vi "Find Var.vi"(8 "error in (no error)":errorcluster, 9 "Tag":string, 10 "Abs_Type Default":refnum<class "Abs_Type.lvclass">, 11 "Var Bus in":refnum<class "Var Bus.lvclass">) -> (0 "error out":errorcluster, 2 "Abs_Type Found":refnum<class "Abs_Type.lvclass">, 3 "Var Bus out":refnum<class "Var Bus.lvclass">)   [LabVIEW 2021, in "Var Bus.lvclass"]
uses:
  Var Bus.lvclass
  LV_Abstract/Source/Abs_Types/Type/Abs_Type.lvclass
  Var Bus.lvclass/Var Bus.ctl
  Properties/Read Var Map.vi
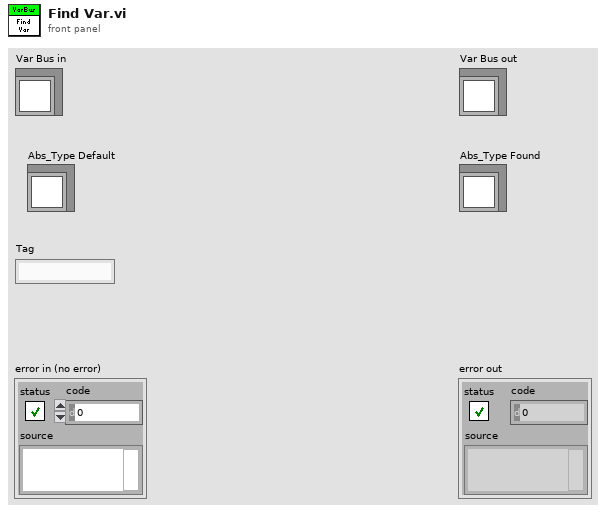
[diagram p1: front panel]
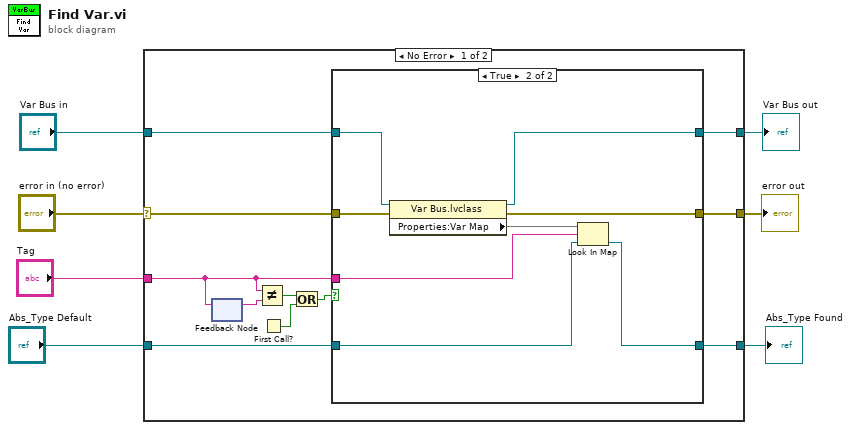
[diagram p0: block diagram]
diagram:
  n1 = case shown="No Error" "error in (no error)" {
    selector: "error in (no error)" -> [w18 w31]
    tunnel: [w15 w31] -> w6
    tunnel: [w14 w30] -> w4
    tunnel: "Var Bus in" -> [w17 w30]
    tunnel: "Tag" -> [w11 _]
    tunnel: [w16 _] -> w2
    tunnel: "Abs_Type Default" -> [w13 _]
    frame No Error {
      n2 = feedback-in #1(w11) -> ()
      n3 = feedback #1() -> (w12:string)  [unwired: 1 in]
      n4 = Not Equal?(x=w11, y=w12) -> (x != y?=w10:bool)
      n5 = First Call?() -> (First Call?: T/F=w8:bool)
      n6 = Or(x=w10, y=w8) -> (x .or. y?=w9:bool)
      n7 = case shown="True" w9 {
        tunnel: w18 -> [w20 w29]
        tunnel: w17 -> [w19 w28]
        tunnel: [w21 w26] -> w16
        tunnel: [w20 w25] -> w15
        tunnel: [w19 w24] -> w14
        tunnel: w13 -> [w21 w23]
        tunnel: w11 -> [_ w22]
        frame False {
        }
        frame True {
          n8 = property class="Var Bus.lvclass"(reference=w28, error in=w29) -> (reference out=w24:refnum<class "Var Bus.lvclass">, error out=w25:errorcluster, "Properties:Var Map"=w27:map{string, refnum<class "Abs_Type.lvclass">})
          n9 = Look In Map(map=w27, key=w22, default value=w23) -> (value=w26:refnum<class "Abs_Type.lvclass">)  [unwired: 1 out]
        }
      }
    }
    frame Error {
    }
  }
  "error out" <- w6
  "Var Bus out" <- w4
  "Abs_Type Found" <- w2
